vi "Cowl_Execute.vi"() -> ()   [LabVIEW 2019]
uses:
  Utility_VIs/Basic_Motor_Modes.ctl
  Globals/Cowl_Globals.vi
panel:
  out "Cowl_Output":dbl
  in  "Kp":dbl
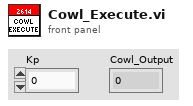
[diagram p1: front panel]
types:
  T1 = typedef "Basic_Motor_Modes.ctl" = enum16{"Percent_Voltage", "Speed_Control", "Position_Control", "Current"}
  T2 = typedef "Cowl_Cluster.ctl" = cluster{"Control_State\n":T3, "Manual_Cowl_%Power":dbl}
  T3 = typedef "Cowl_States.ctl" = enum16{"Manual_%VBus", "GoToAngle"}
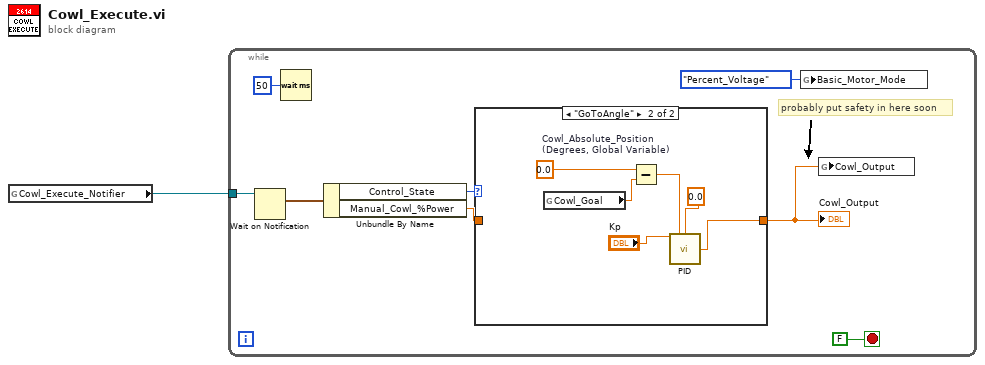
[diagram p0: block diagram]
diagram:
  n1 = global read "Cowl_Globals.vi" "Cowl_Execute_Notifier"() -> (w1:refnum<notifier>)
  n2 = while {
    tunnel: w1 -> [w7]
    stop <- FALSE stop-if-true
    # "probably put safety in here soon"
    n3 = Wait on Notification(notifier=w7) -> (notification=w6:T2)  [unwired: 3 in, 3 out]
    n4 = Wait (ms)(milliseconds to wait=u32 50) -> ()  [unwired: 1 out]
    n5 = Unbundle By Name(w6) -> ("Control_State"=w5:T3, "Manual_Cowl_%Power"=w4:dbl)
    n6 = case shown="\"GoToAngle\"" w5 {
      tunnel: w4 -> [w10 _]
      tunnel: [w10 w16] -> w3
      frame "Manual_%VBus", Default {
      }
      frame "GoToAngle" {
        w13 = 0.0  # Cowl_Absolute_Position (Degrees, Global Variable)
        n7 = global read "Cowl_Globals.vi" "Cowl_Goal"() -> (w14:dbl)
        n8 = Subtract(x=w13, y=w14) -> (x-y=w12:dbl)
        n9 = call "PID.vi"("Kp"="Kp", "Process Variable"=w12, "Goal"=0.0) -> ("Command"=w16:dbl)  [unwired: 10 in, 2 out]
      }
    }
    "Cowl_Output" <- w3
    n10 = global write "Cowl_Globals.vi" "Basic_Motor_Mode"(Basic_Motor_Modes."Percent_Voltage" ("Basic_Motor_Mode")) -> ()
    n11 = global write "Cowl_Globals.vi" "Cowl_Output"(w3) -> ()
  }
